vi "Autonomous Independent.vi"() -> ()   [LabVIEW 2018]
doc: "This VI is called when autonomous begins, and will automatically be terminated when autonomous ends. You can carry out timed or sensor driven robot movement independently without needing to return to the caller."
uses:
  <vilib>/Rock Robotics/WPI/Utilities/WPI_GetSetVariantRefNum.vi
  <vilib>/Rock Robotics/Network Tables/NT Read String.vi
  <vilib>/Rock Robotics/Network Tables/NT Write Numeric Array.vi
  <vilib>/Rock Robotics/WPI/RobotDrive/WPI_RobotDriveArcadeDrive_Standard(NoSaturation).vi
panel:
  out "Current Movement, for debugging":T1 {"Y Joystick Value" scale=1.0..-1.0; "X Joystick Value" scale=-1.0..1.0}
  in  "Array of robot movements":T2(array[cluster])=[{"X Joystick Value"=0.39393939393939403, "Y Joystick Value"=0.0, "Delay (sec)"=1.0, "Movement Name"="turn"}, {"X Joystick Value"=-0.3737373737373737, "Y Joystick Value"=0.0, "Delay (sec)"=1.0, "Movement Name"="turn back"}] {"Y Joystick Value" scale=1.0..-1.0; "X Joystick Value" scale=-1.0..1.0}
  # "Be sure to right-click and choose Data Operations>>Make Current Value default if you want to save the array values with the VI"
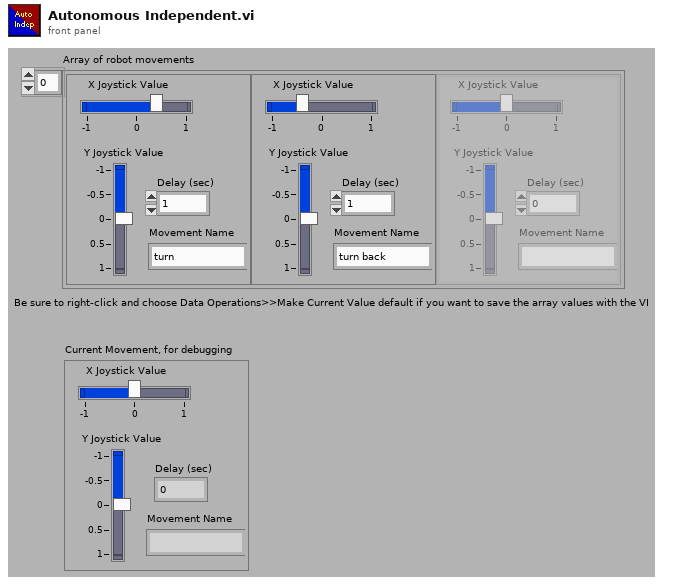
[diagram p1: front panel]
types:
  T1 = cluster{"X Joystick Value":dbl, "Y Joystick Value":dbl, "Delay (sec)":dbl, "Movement Name":string}
  T2 = cluster{"X Joystick Value":dbl, "Y Joystick Value":dbl, "Delay (sec)":dbl, "Movement Name":string}[]
  T3 = typedef "WPI_JoystickDevRef.ctl" = cluster{"Device":T4}
  T4 = typedef "WPI_JoystickDeviceEnum.ctl" = enum16{"USB 0", "USB 1", "USB 2", "USB 3", "USB 4", "USB 5"}
  T5 = typedef "WPI_RobotDriveDevRef.ctl" = cluster{"DevStatus":errorcluster, "Motors[]":T6[], "Square Inputs":bool, "Max Output":dbl}
  T6 = typedef "WPI_MotorControlDeviceRef.ctl" = cluster{"DeviceStatus":errorcluster, "Type":T7, "PWM":cluster{"PWM Channel":T8, "DeadBand":T9}, "CAN":cluster{"Device Number":u8, "SetOutput VI Ref":variant, "GetOutput VI Ref":variant, "Enable VI Ref":variant, "Disable VI Ref":variant, "Data":variant}, "Invert":bool, "DIO PWM":cluster{"PWM \"Enable\" Channel":T8, "DIOChannel":T10, "PWM Rate":dbl}}
  T7 = typedef "WPI_MotorControlType.ctl" = enum16{"PWM", "CAN", "DIO PWM"}
  T8 = typedef "FPGA_DIOPWMChannel.ctl" = enum8{"PWM 0", "PWM 1", "PWM 2", "PWM 3", "PWM 4", "PWM 5", "PWM 6", "PWM 7", "PWM 8", "PWM 9", "PWM MXP 0", "PWM MXP 1", "PWM MXP 2", "PWM MXP 3", "PWM MXP 4", "PWM MXP 5", "PWM MXP 6", "PWM MXP 7", "PWM MXP 8", "PWM MXP 9", "Invalid"}
  T9 = typedef "WPI_PWMDeadband.ctl" = cluster{"Name":string, "maxPositivePwm":i32, "minPositivePwm":i32, "centerPwm":i32, "maxNegativePwm":i32, "minNegativePwm":i32, "angularRange":u16}
  T10 = typedef "FPGA_DIOChannel.ctl" = enum8{"DIO 0", "DIO 1", "DIO 2", "DIO 3", "DIO 4", "DIO 5", "DIO 6", "DIO 7", "DIO 8", "DIO 9", "DIO MXP 0", "DIO MXP 1", "DIO MXP 2", "DIO MXP 3", "DIO MXP 4", "DIO MXP 5", "DIO MXP 6", "DIO MXP 7", "DIO MXP 8", "DIO MXP 9", "DIO MXP 10", "DIO MXP 11", "DIO MXP 12", "DIO MXP 13", "DIO MXP 14", "DIO MXP 15", "SPI Port CS1", "SPI Port CS2", "SPI Port CS3", "SPI Port MISO", "SPI Port MOSI", "Invalid"}
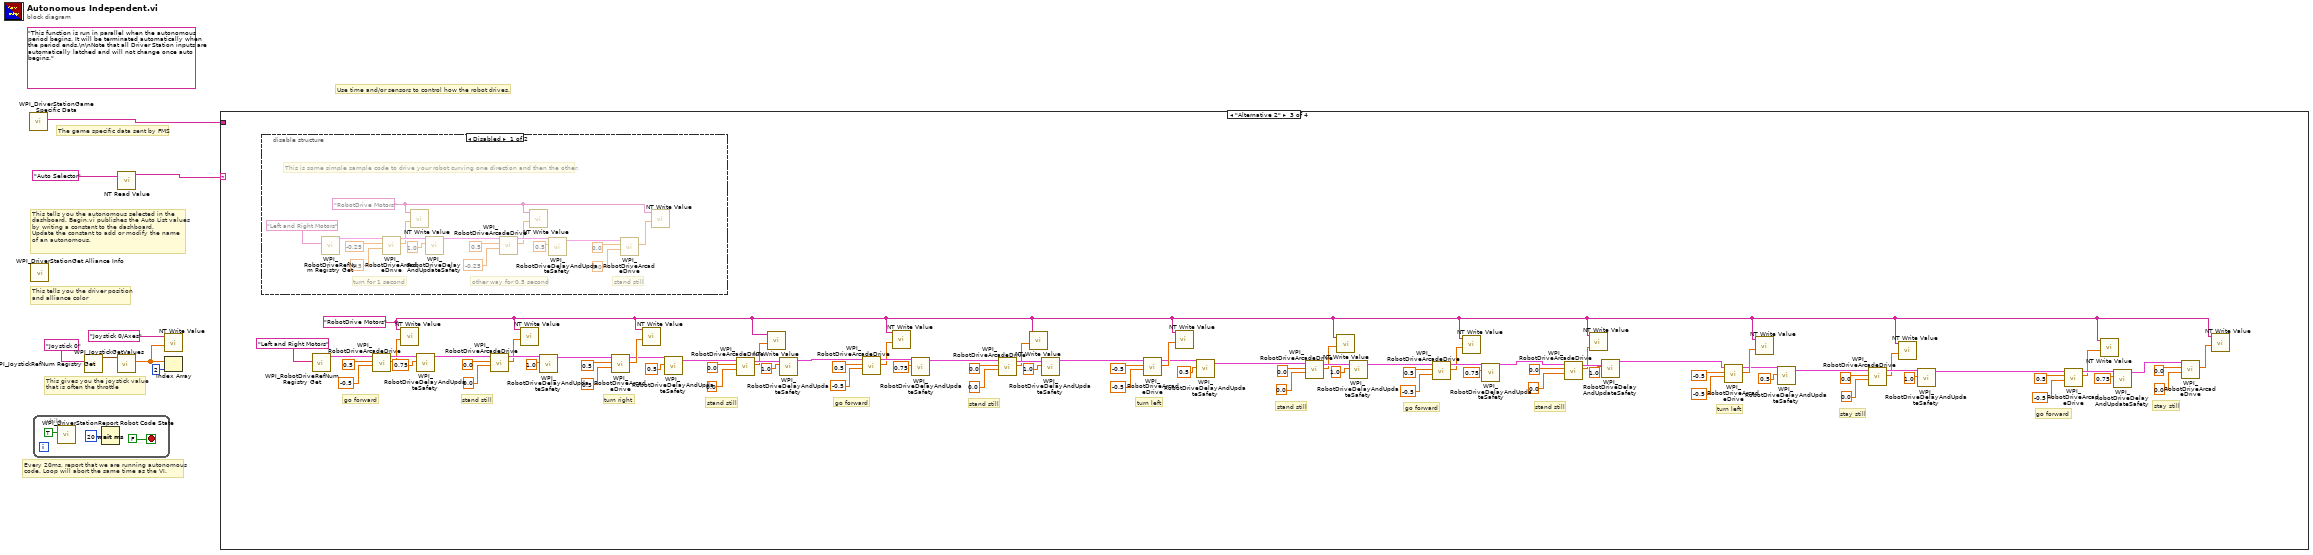
[diagram p0: block diagram]
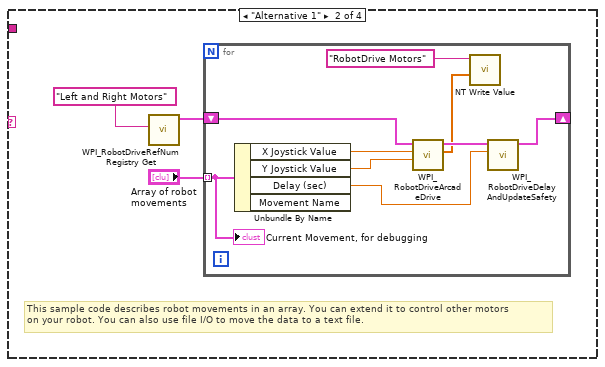
[diagram p3: hidden frame]
diagram:
  (unwired) "This function is run in parallel when the autonomous period begins. It will be terminated automatically when the period ends.\n\nNote that all Driver Station inputs are automatically latched and will not change once auto begins."
  # "The game specific data sent by FMS"
  # "This tells you the autonomous selected in the \ndashboard. Begin.vi publishes the Auto List values\nby writing a constant to the dashboard.\nUpdate the constant to add or modify the name\nof an autonomous."
  # "Every 20ms, report that we are running autonomous\ncode. Loop will abort the same time as the VI."
  # "This gives you the joystick value\nthat is often the throttle"
  # "Use time and/or sensors to control how the robot drives."
  # "This tells you the driver position\nand alliance color"
  n1 = call <vilib>:"WPI_DriverStationGame Specific Data.vi"() -> ("Game Specific Data"=w1:string)  [unwired: 11 in]
  n2 = call <vilib>:"WPI_DriverStationGet Alliance Info.vi"() -> ()  [unwired: 12 out]
  n3 = while {
    stop <- FALSE stop-if-true
    n4 = call <vilib>:"WPI_DriverStationReport Robot Code State.vi"("Autonomous"=TRUE) -> ()  [unwired: 10 in, 1 out]
    n5 = Wait (ms)(milliseconds to wait=u32 20) -> ()  [unwired: 1 out]
  }
  n6 = call <vilib>:"WPI_JoystickRefNum Registry Get.vi"("refnum name"="Joystick 0") -> ("JoystickDevRef"=w7:T3)  [unwired: 1 in, 9 out]
  n7 = call <vilib>:"WPI_JoystickGetValues.vi"("JoystickDevRef"=w7) -> ("Axes"=w3:dbl[])  [unwired: 6 in, 4 out]
  n8 = call-poly <vilib>:"NT Read Value.vi"("Name"="Auto Selector") -> ("String"=w4:string)  [unwired: 9 in, 1 out]
  n9 = call-poly <vilib>:"NT Write Value.vi"("Numeric Array"=w3, "Name"="Joystick 0/Axes") -> ()  [unwired: 9 in, 1 out]
  n10 = Index Array(array=w3, index=2) -> ()  [unwired: 1 out]
  n11 = case shown="\"Alternative 2\"" w4 {
    tunnel: w1 -> [_ _ _ _]
    frame Default {
      # "You can put your main auto here, or you can right-click on the case and make any\nother frame be the default case."
      # "This is the frame that will execute if no selection is made, or if it is not recognized"
    }
    frame "Alternative 1" {
      # "This sample code describes robot movements in an array. You can extend it to control other motors\non your robot. You can also use file I/O to move the data to a text file."
      n12 = call <vilib>:"WPI_RobotDriveRefNum Registry Get.vi"("refnum name"="Left and Right Motors") -> ("RobotDriveDevRef"=w13:T5)  [unwired: 1 in, 9 out]
      n13 = for {
        shift-right: [w21] -> _
        shift-left: w13 -> [w22]
        tunnel: "Array of robot movements" -> [w17] mode=indexing
        n14 = Unbundle By Name(w17) -> ("X Joystick Value"=w20:dbl, "Y Joystick Value"=w19:dbl, "Delay (sec)"=w18:dbl)  [unwired: 1 out]
        n15 = call-poly <vilib>:"WPI_RobotDriveArcadeDrive.vi"("Y axis value"=w19, "X axis value"=w20, "RobotDriveDevRef"=w22) -> ("Motor Values"=w15:dbl[], "RobotDriveDevRef"=w23:T5)  [unwired: 1 in, 6 out]
        n16 = call-poly <vilib>:"NT Write Value.vi"("Numeric Array"=w15, "Name"="RobotDrive Motors") -> ()  [unwired: 9 in, 1 out]
        n17 = call <vilib>:"WPI_RobotDriveDelayAndUpdateSafety.vi"("Delay (s)"=w18, "RobotDriveDevRef"=w23) -> ("RobotDriveDevRef 2"=w21:T5)  [unwired: 8 in, 1 out]
        "Current Movement, for debugging" <- w17
      }
    }
    frame "Alternative 2" {
      w25 = "RobotDrive Motors" ("Name")
      # "stay still"
      # "go forward"
      # "stay still"
      # "turn left"
      # "stand still"
      # "go forward"
      # "stand still"
      # "turn left"
      # "stand still"
      # "go forward"
      # "stand still"
      # "turn right"
      # "stand still"
      # "go forward"
      n18 = disable-structure shown="Disabled" {
        frame Disabled {
          w109 = "RobotDrive Motors" ("Name")
          # "This is some simple sample code to drive your robot curving one direction and then the other."
          # "stand still"
          # "other way for 0.5 second"
          # "turn for 1 second"
          n19 = call <vilib>:"WPI_RobotDriveRefNum Registry Get.vi"("refnum name"="Left and Right Motors") -> ("RobotDriveDevRef"=w125:T5)  [unwired: 1 in, 9 out]
          n20 = call-poly <vilib>:"WPI_RobotDriveArcadeDrive.vi"("Y axis value"=0.5 ("X axis value"), "X axis value"=-0.25, "RobotDriveDevRef"=w125) -> ("Motor Values"=w108:dbl[], "RobotDriveDevRef"=w118:T5)  [unwired: 1 in, 6 out]
          n21 = call-poly <vilib>:"NT Write Value.vi"("Numeric Array"=w108, "Name"=w109) -> ()  [unwired: 9 in, 1 out]
          n22 = call <vilib>:"WPI_RobotDriveDelayAndUpdateSafety.vi"("Delay (s)"=1.0, "RobotDriveDevRef"=w118) -> ("RobotDriveDevRef 2"=w119:T5)  [unwired: 8 in, 1 out]
          n23 = call-poly <vilib>:"WPI_RobotDriveArcadeDrive.vi"("Y axis value"=-0.25 ("X axis value"), "X axis value"=0.5, "RobotDriveDevRef"=w119) -> ("Motor Values"=w110:dbl[], "RobotDriveDevRef"=w120:T5)  [unwired: 1 in, 6 out]
          n24 = call-poly <vilib>:"NT Write Value.vi"("Numeric Array"=w110, "Name"=w109) -> ()  [unwired: 9 in, 1 out]
          n25 = call <vilib>:"WPI_RobotDriveDelayAndUpdateSafety.vi"("Delay (s)"=0.5, "RobotDriveDevRef"=w120) -> ("RobotDriveDevRef 2"=w121:T5)  [unwired: 8 in, 1 out]
          n26 = call-poly <vilib>:"WPI_RobotDriveArcadeDrive.vi"("Y axis value"=0.0 ("X axis value"), "X axis value"=0.0, "RobotDriveDevRef"=w121) -> ("Motor Values"=w111:dbl[])  [unwired: 1 in, 7 out]
          n27 = call-poly <vilib>:"NT Write Value.vi"("Numeric Array"=w111, "Name"=w109) -> ()  [unwired: 9 in, 1 out]
        }
        frame Enabled {
        }
      }
      n28 = call <vilib>:"WPI_RobotDriveRefNum Registry Get.vi"("refnum name"="Left and Right Motors") -> ("RobotDriveDevRef"=w107:T5)  [unwired: 1 in, 9 out]
      n29 = call-poly <vilib>:"WPI_RobotDriveArcadeDrive.vi"("Y axis value"=-0.5 ("X axis value"), "X axis value"=0.5, "RobotDriveDevRef"=w107) -> ("Motor Values"=w91:dbl[], "RobotDriveDevRef"=w100:T5)  [unwired: 1 in, 6 out]
      n30 = call-poly <vilib>:"NT Write Value.vi"("Numeric Array"=w91, "Name"=w25) -> ()  [unwired: 9 in, 1 out]
      n31 = call <vilib>:"WPI_RobotDriveDelayAndUpdateSafety.vi"("Delay (s)"=0.75, "RobotDriveDevRef"=w100) -> ("RobotDriveDevRef 2"=w101:T5)  [unwired: 8 in, 1 out]
      n32 = call-poly <vilib>:"WPI_RobotDriveArcadeDrive.vi"("Y axis value"=0.0 ("X axis value"), "X axis value"=0.0, "RobotDriveDevRef"=w101) -> ("Motor Values"=w92:dbl[], "RobotDriveDevRef"=w102:T5)  [unwired: 1 in, 6 out]
      n33 = call-poly <vilib>:"NT Write Value.vi"("Numeric Array"=w92, "Name"=w25) -> ()  [unwired: 9 in, 1 out]
      n34 = call <vilib>:"WPI_RobotDriveDelayAndUpdateSafety.vi"("Delay (s)"=1.0, "RobotDriveDevRef"=w102) -> ("RobotDriveDevRef 2"=w103:T5)  [unwired: 8 in, 1 out]
      n35 = call-poly <vilib>:"WPI_RobotDriveArcadeDrive.vi"("Y axis value"=0.5 ("X axis value"), "X axis value"=0.5, "RobotDriveDevRef"=w103) -> ("Motor Values"=w93:dbl[], "RobotDriveDevRef"=w90:T5)  [unwired: 1 in, 6 out]
      n36 = call-poly <vilib>:"NT Write Value.vi"("Numeric Array"=w93, "Name"=w25) -> ()  [unwired: 9 in, 1 out]
      n37 = call <vilib>:"WPI_RobotDriveDelayAndUpdateSafety.vi"("Delay (s)"=0.5, "RobotDriveDevRef"=w90) -> ("RobotDriveDevRef 2"=w83:T5)  [unwired: 8 in, 1 out]
      n38 = call-poly <vilib>:"WPI_RobotDriveArcadeDrive.vi"("Y axis value"=0.0 ("X axis value"), "X axis value"=0.0, "RobotDriveDevRef"=w83) -> ("Motor Values"=w84:dbl[], "RobotDriveDevRef"=w87:T5)  [unwired: 1 in, 6 out]
      n39 = call-poly <vilib>:"NT Write Value.vi"("Numeric Array"=w84, "Name"=w25) -> ()  [unwired: 9 in, 1 out]
      n40 = call <vilib>:"WPI_RobotDriveDelayAndUpdateSafety.vi"("Delay (s)"=1.0, "RobotDriveDevRef"=w87) -> ("RobotDriveDevRef 2"=w77:T5)  [unwired: 8 in, 1 out]
      n41 = call-poly <vilib>:"WPI_RobotDriveArcadeDrive.vi"("Y axis value"=-0.5 ("X axis value"), "X axis value"=0.5, "RobotDriveDevRef"=w77) -> ("Motor Values"=w78:dbl[], "RobotDriveDevRef"=w81:T5)  [unwired: 1 in, 6 out]
      n42 = call-poly <vilib>:"NT Write Value.vi"("Numeric Array"=w78, "Name"=w25) -> ()  [unwired: 9 in, 1 out]
      n43 = call <vilib>:"WPI_RobotDriveDelayAndUpdateSafety.vi"("Delay (s)"=0.75, "RobotDriveDevRef"=w81) -> ("RobotDriveDevRef 2"=w71:T5)  [unwired: 8 in, 1 out]
      n44 = call-poly <vilib>:"WPI_RobotDriveArcadeDrive.vi"("Y axis value"=0.0 ("X axis value"), "X axis value"=0.0, "RobotDriveDevRef"=w71) -> ("Motor Values"=w72:dbl[], "RobotDriveDevRef"=w75:T5)  [unwired: 1 in, 6 out]
      n45 = call-poly <vilib>:"NT Write Value.vi"("Numeric Array"=w72, "Name"=w25) -> ()  [unwired: 9 in, 1 out]
      n46 = call <vilib>:"WPI_RobotDriveDelayAndUpdateSafety.vi"("Delay (s)"=1.0, "RobotDriveDevRef"=w75) -> ("RobotDriveDevRef 2"=w65:T5)  [unwired: 8 in, 1 out]
      n47 = call-poly <vilib>:"WPI_RobotDriveArcadeDrive.vi"("Y axis value"=-0.5 ("X axis value"), "X axis value"=-0.5, "RobotDriveDevRef"=w65) -> ("Motor Values"=w68:dbl[], "RobotDriveDevRef"=w67:T5)  [unwired: 1 in, 6 out]
      n48 = call-poly <vilib>:"NT Write Value.vi"("Numeric Array"=w68, "Name"=w25) -> ()  [unwired: 9 in, 1 out]
      n49 = call <vilib>:"WPI_RobotDriveDelayAndUpdateSafety.vi"("Delay (s)"=0.5, "RobotDriveDevRef"=w67) -> ("RobotDriveDevRef 2"=w59:T5)  [unwired: 8 in, 1 out]
      n50 = call-poly <vilib>:"WPI_RobotDriveArcadeDrive.vi"("Y axis value"=0.0 ("X axis value"), "X axis value"=0.0, "RobotDriveDevRef"=w59) -> ("Motor Values"=w60:dbl[], "RobotDriveDevRef"=w63:T5)  [unwired: 1 in, 6 out]
      n51 = call-poly <vilib>:"NT Write Value.vi"("Numeric Array"=w60, "Name"=w25) -> ()  [unwired: 9 in, 1 out]
      n52 = call <vilib>:"WPI_RobotDriveDelayAndUpdateSafety.vi"("Delay (s)"=1.0, "RobotDriveDevRef"=w63) -> ("RobotDriveDevRef 2"=w53:T5)  [unwired: 8 in, 1 out]
      n53 = call-poly <vilib>:"WPI_RobotDriveArcadeDrive.vi"("Y axis value"=-0.5 ("X axis value"), "X axis value"=0.5, "RobotDriveDevRef"=w53) -> ("Motor Values"=w54:dbl[], "RobotDriveDevRef"=w57:T5)  [unwired: 1 in, 6 out]
      n54 = call-poly <vilib>:"NT Write Value.vi"("Numeric Array"=w54, "Name"=w25) -> ()  [unwired: 9 in, 1 out]
      n55 = call <vilib>:"WPI_RobotDriveDelayAndUpdateSafety.vi"("Delay (s)"=0.75, "RobotDriveDevRef"=w57) -> ("RobotDriveDevRef 2"=w47:T5)  [unwired: 8 in, 1 out]
      n56 = call-poly <vilib>:"WPI_RobotDriveArcadeDrive.vi"("Y axis value"=0.0 ("X axis value"), "X axis value"=0.0, "RobotDriveDevRef"=w47) -> ("Motor Values"=w48:dbl[], "RobotDriveDevRef"=w51:T5)  [unwired: 1 in, 6 out]
      n57 = call-poly <vilib>:"NT Write Value.vi"("Numeric Array"=w48, "Name"=w25) -> ()  [unwired: 9 in, 1 out]
      n58 = call <vilib>:"WPI_RobotDriveDelayAndUpdateSafety.vi"("Delay (s)"=1.0, "RobotDriveDevRef"=w51) -> ("RobotDriveDevRef 2"=w41:T5)  [unwired: 8 in, 1 out]
      n59 = call-poly <vilib>:"WPI_RobotDriveArcadeDrive.vi"("Y axis value"=-0.5 ("X axis value"), "X axis value"=-0.5, "RobotDriveDevRef"=w41) -> ("Motor Values"=w44:dbl[], "RobotDriveDevRef"=w43:T5)  [unwired: 1 in, 6 out]
      n60 = call-poly <vilib>:"NT Write Value.vi"("Numeric Array"=w44, "Name"=w25) -> ()  [unwired: 9 in, 1 out]
      n61 = call <vilib>:"WPI_RobotDriveDelayAndUpdateSafety.vi"("Delay (s)"=0.5, "RobotDriveDevRef"=w43) -> ("RobotDriveDevRef 2"=w35:T5)  [unwired: 8 in, 1 out]
      n62 = call-poly <vilib>:"WPI_RobotDriveArcadeDrive.vi"("Y axis value"=0.0 ("X axis value"), "X axis value"=0.0, "RobotDriveDevRef"=w35) -> ("Motor Values"=w36:dbl[], "RobotDriveDevRef"=w39:T5)  [unwired: 1 in, 6 out]
      n63 = call-poly <vilib>:"NT Write Value.vi"("Numeric Array"=w36, "Name"=w25) -> ()  [unwired: 9 in, 1 out]
      n64 = call <vilib>:"WPI_RobotDriveDelayAndUpdateSafety.vi"("Delay (s)"=1.0, "RobotDriveDevRef"=w39) -> ("RobotDriveDevRef 2"=w29:T5)  [unwired: 8 in, 1 out]
      n65 = call-poly <vilib>:"WPI_RobotDriveArcadeDrive.vi"("Y axis value"=-0.5 ("X axis value"), "X axis value"=0.5, "RobotDriveDevRef"=w29) -> ("Motor Values"=w30:dbl[], "RobotDriveDevRef"=w33:T5)  [unwired: 1 in, 6 out]
      n66 = call-poly <vilib>:"NT Write Value.vi"("Numeric Array"=w30, "Name"=w25) -> ()  [unwired: 9 in, 1 out]
      n67 = call <vilib>:"WPI_RobotDriveDelayAndUpdateSafety.vi"("Delay (s)"=0.75, "RobotDriveDevRef"=w33) -> ("RobotDriveDevRef 2"=w24:T5)  [unwired: 8 in, 1 out]
      n68 = call-poly <vilib>:"WPI_RobotDriveArcadeDrive.vi"("Y axis value"=0.0 ("X axis value"), "X axis value"=0.0, "RobotDriveDevRef"=w24) -> ("Motor Values"=w26:dbl[])  [unwired: 1 in, 7 out]
      n69 = call-poly <vilib>:"NT Write Value.vi"("Numeric Array"=w26, "Name"=w25) -> ()  [unwired: 9 in, 1 out]
    }
    frame "Your Turn" {
    }
  }
